vi "LAS-CTS_LaserEnergyHistogram.vi"() -> ()   [LabVIEW 2024]
uses:
  <vilib>/Platform/TimedLoop/XDataNode/timing_clust.ctl
  <vilib>/Platform/TimedLoop/XDataNode/nitl_modes.ctl
  <vilib>/Platform/TimedLoop/XDataNode/wakeup.ctl
  <vilib>/Utility/file.llb/Write Delimited Spreadsheet (DBL).vi
  <vilib>/platform/TimedLoop/XDataNode/XDataNode.xnode
  <vilib>/Platform/TimedLoop/XDataNode/XDNodeRunTimeDep.lvlib
  <vilib>/Analysis/NI_AALBase.lvlib
panel:
  out "standard deviation":dbl format="%0.2f"
  out "mean":dbl format="%0.2f"
  out "Waveform Graph":dbl[](graph)
  out "# of measurements":i32
  out "Histogram Graph":T1(graph)
  in  "File Name":path
  in  "Folder Name":path
  in  "Rep Rate":u16(ring)=1 items=["20 Hz"=1, "10 Hz"=2, "5 Hz"=4, "4 Hz"=5, "2 Hz"=10, "1 Hz"=20]
  in  "Energy Meter":refnum<visa-resource-name>
  in  "# of Pulses":i32
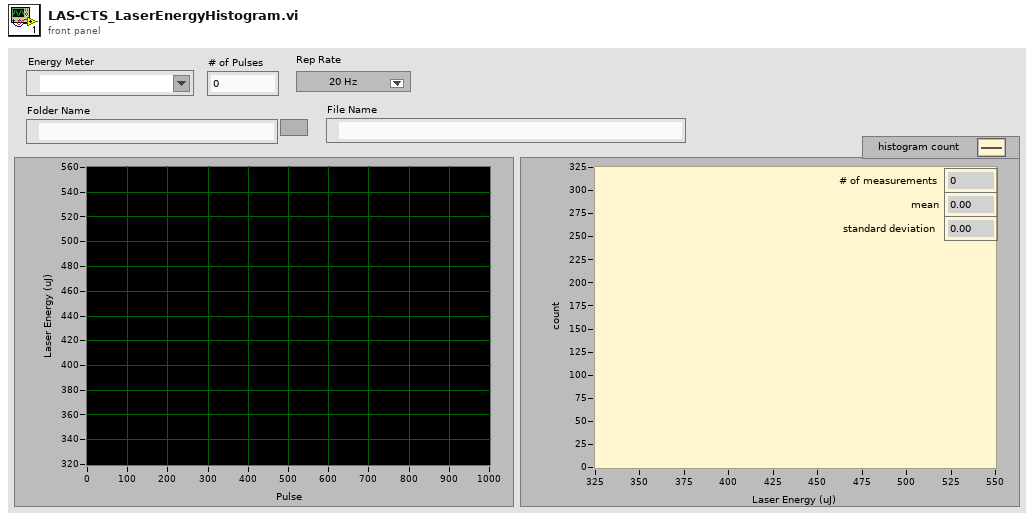
[diagram p1: front panel]
types:
  T1 = cluster{"X Values":dbl[], "Histogram: h(x)":i32[]}
  T2 = typedef "LabVIEWHTTPClient.lvlib/ClientHandle.ctl" = refnum<k1>
  T3 = typedef "XDNodeRunTimeDep.lvlib/timing_clust.ctl" = cluster{"Expected End [f-1]":u64, "Actual End [f-1]":u64, "Finished Late? [f-1]":bool, "Expected End [i-1]":u64, "Actual End [i-1]":u64, "Finished Late? [i-1]":bool, "Expected Start [i]":u64, "Actual Start [i]":u64, "Expected Start [f]":u64, "Actual Start [f]":u64, "Source Name":string, "Structure Name":string, "Period":i64, "Deadline":i64, "Offset":i64, "Start":i64, "Priority":i32, "Timeout":i32, "Mode":T4, "Wakeup Reason":T5, "Error":errorcluster, "Source Type":string, "Secondary Source Type":string, "Global End Time":u64, "Global Start Time":u64, "Frame Duration":u64, "Iteration Duration":u64, "Assigned CPU":i32, "I/O Scan Engine Mode":u32}
  T4 = typedef "XDNodeRunTimeDep.lvlib/nitl_modes.ctl" = enum32{"No Change", "Process missed periods, maintain original phase", "Discard missed periods, maintain original phase", "Process missed periods, ignore original phase", "Discard missed periods, ignore original phase"}
  T5 = typedef "XDNodeRunTimeDep.lvlib/wakeup.ctl" = enum32{"Normal", "Aborted", "Asynchronous wakeup", "Timing source error", "Timed loop error", "Timeout"}
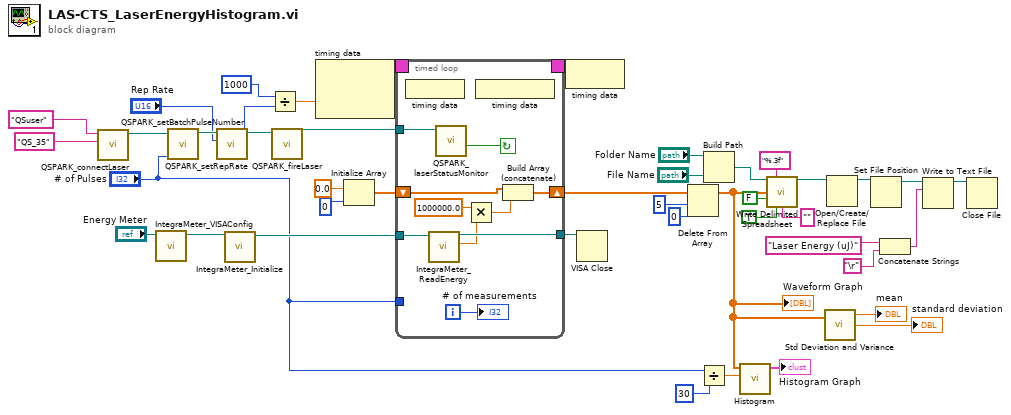
[diagram p0: block diagram]
diagram:
  n1 = call "QSPARK_connectLaser.vi"("password"="QS_35", "username"="QSuser") -> ("client handle out"=w41:T2)  [unwired: 9 in]
  n2 = call "IntegraMeter_VISAConfig.vi"("VISA resource name"="Energy Meter") -> ("reference out"=w43:refnum<visa-resource-name>)  [unwired: 9 in, 1 out]
  n3 = call "QSPARK_setBatchPulseNumber.vi"("Number of Pulses"="# of Pulses", "client handle"=w41) -> ("client handle out"=w36:T2)  [unwired: 9 in]
  n4 = call "QSPARK_setRepRate.vi"("Rep Rate"="Rep Rate", "client handle"=w36) -> ("Rep Rate (Hz)"=w9:i32, "client handle out"=w33:T2)  [unwired: 8 in]
  n5 = call "IntegraMeter_Initialize.vi"("VISA resource name"=w43) -> ("VISA resource name out"=w30:refnum<visa-resource-name>)  [unwired: 9 in, 1 out]
  n6 = Divide(x=1000, y=w9) -> (x/y=w35:dbl)
  n7 = call "QSPARK_fireLaser.vi"("client handle"=w33) -> ("client handle out"=w10:T2)  [unwired: 10 in]
  n8 = node-c288(w35) -> (w38:T3)  [unwired: 1 in]
  n9 = Initialize Array(0.0 ("element"), 0 ("dimension size")) -> (w29:dbl[])
  n10 = timed-loop {
    timing: w38 -> [_]
    timing-out: [_] -> w37
    tunnel: w30 -> [w53]
    shift-right: [w52] -> w5
    shift-left: w29 -> [w51]
    tunnel: [w50] -> w28
    tunnel: "# of Pulses" -> [_]
    tunnel: w10 -> [w46]
    i -> [w44]
    stop <- w45 continue-if-true
    n11 = node-c288() -> ()  [unwired: 1 in]
    n12 = call "IntegraMeter_ReadEnergy.vi"("VISA resource name"=w53) -> ("Laser Energy (J)"=w48:dbl, "VISA resource name out"=w50:refnum<visa-resource-name>)  [unwired: 8 in, 1 out]
    n13 = call "QSPARK_laserStatusMonitor.vi"("client handle"=w46) -> ("laser on?"=w45:bool)  [unwired: 8 in, 2 out]
    n14 = Multiply(x=1000000.0, y=w48) -> (x*y=w49:dbl)
    n15 = node-c288() -> ()  [unwired: 1 out]
    n16 = Build Array (concatenate)(w51, w49) -> (w52:dbl[])
    "# of measurements" <- w44
  }
  n17 = node-c288(w37) -> ()
  n18 = VISA Close(VISA resource name=w28) -> ()  [unwired: 1 in, 1 out]
  n19 = Delete From Array(array=w5, length=5, index=0) -> (array with subset deleted=w3:dbl[])  [unwired: 1 out]
  "Waveform Graph" <- w3
  n20 = Divide(x="# of Pulses", y=30) -> (x/y=w14:dbl)
  n21 = Build Path(base path="Folder Name", name or relative path="File Name") -> (appended path=w22:path)
  n22 = call <vilib>:"Histogram.vi"("intervals"=w14, "X"=w3) -> ("Histogram Graph"=→"Histogram Graph":T1)  [unwired: 6 in, 3 out]
  n23 = call-poly <vilib>:"Write Delimited Spreadsheet.vi"("file path (dialog if empty)"=w22, "format (%.3f)"="%.3f", "1D data"=w3, "append to file? (new file:F)"=FALSE, "transpose? (no:F)"=TRUE, "delimiter (\\t)"="" ("delimiter (\\t)")) -> ("new file path (Not A Path if cancelled)"=w21:path)  [unwired: 8 in, 1 out]
  n24 = call <vilib>:"Std Deviation and Variance.vi"("X"=w3) -> ("mean"=→"mean":dbl, "standard deviation"=→"standard deviation":dbl)  [unwired: 1 in, 1 out]
  n25 = Open/Create/Replace File(file path (use dialog)=w21) -> (refnum out=w20:refnum<file>)  [unwired: 5 in, 2 out]
  n26 = Set File Position(refnum=w20) -> (refnum out=w19:refnum<file>)  [unwired: 3 in, 1 out]
  n27 = Concatenate Strings("Laser Energy (uJ)", "\r") -> (w16:string)
  n28 = Write to Text File(file (use dialog)=w19, text=w16) -> (refnum out=w15:refnum<file>)  [unwired: 2 in, 2 out]
  n29 = Close File(refnum=w15) -> ()  [unwired: 1 in, 2 out]
